vi "PH_PSDBWriter.Wrap Numeric Data.vi"(1 "Unit Array":string[](array[string]), 2 "Data Array":dbl[](array[numeric]), 3 "Name Array":string[](array[string]), 4 "Name Prefix":string) -> (0 "PSDB Numeric Data Array":T1[](array[typedef]))   [LabVIEW 2014, in "PH_PSDBWriter.lvlib"]
uses:
  PH_PSDBWriter.lvlib
  PH_PSDBWriter.Numeric dataset.ctl
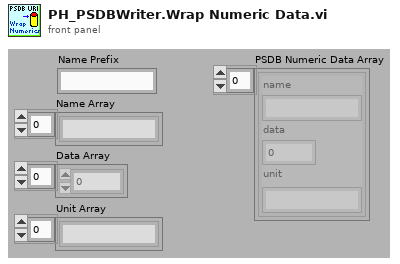
[diagram p1: front panel]
types:
  T1 = typedef "PH_PSDBWriter.lvlib/PH_PSDBWriter.Numeric dataset.ctl" = cluster{"name":string, "data":dbl, "unit":string}
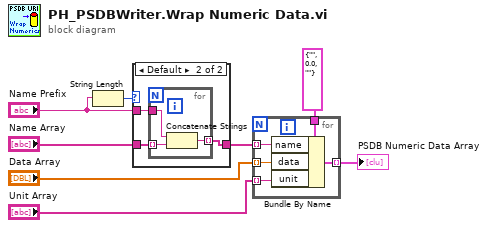
[diagram p0: block diagram]
diagram:
  n1 = String Length(string="Name Prefix") -> (length=w4:i32)
  n2 = case shown="Default" w4 {
    tunnel: "Name Array" -> [w9 w12]
    tunnel: [w9 w10] -> w1
    tunnel: "Name Prefix" -> [_ w11]
    frame 0 {
    }
    frame Default {
      n3 = for {
        tunnel: w12 -> [w15] mode=indexing
        tunnel: w11 -> [w14]
        tunnel: [w13] -> w10 mode=indexing
        n4 = Concatenate Strings(w14, w15) -> (w13:string)
      }
    }
  }
  n5 = for {
    tunnel: T1 {"name"="", "data"=0.0, "unit"=""} ("new element/subarray") -> [w20]
    tunnel: [w19] -> w6 mode=indexing
    tunnel: "Unit Array" -> [w18] mode=indexing
    tunnel: w1 -> [w16] mode=indexing
    tunnel: "Data Array" -> [w17] mode=indexing
    n6 = Bundle By Name(cluster=w20, "name"=w16, "data"=w17, "unit"=w18) -> (w19:T1)
  }
  "PSDB Numeric Data Array" <- w6
